vi "Test Quaternion Average.vi"(11 "Test Case In":refnum<class "03_AR.lvclass">) -> (0 "error out":errorcluster, 3 "Test Case Out":refnum<class "03_AR.lvclass">)   [LabVIEW 2020, in "test.lvlib" / "03_AR.lvclass"]
uses:
  03_AR.lvclass
  C:/Program Files (x86)/National Instruments/LabVIEW 2026/vi.lib/Astemes/LUnit/Test Case.lvclass
  ar/Quaternion.ctl
  <vilib>/Astemes/LUnit/Test Case.lvclass/Test Case.ctl
  4993e8ee-a06a-463a-9684-69129f64d5ce.vi
  <vilib>/Astemes/LUnit/Core/LUnit Test Case/Private/Append Pass Result.vi
  <vilib>/Astemes/LUnit/Core/LUnit Test Case/Private/Append Fail Result.vi
  4993e8ee-a06a-463a-9684-69129f64d5ce.vi/9c5d11cd-9439-4240-a1ee-d9baace9c924.vi
  <vilib>/Astemes/LUnit/Core/LUnit Test Case/Private/Run In UI.vi
  <vilib>/Utility/error.llb/Clear Errors.vi
  <vilib>/Utility/error.llb/Error Cluster From Error Code.vi
  ar/ar.lvlib
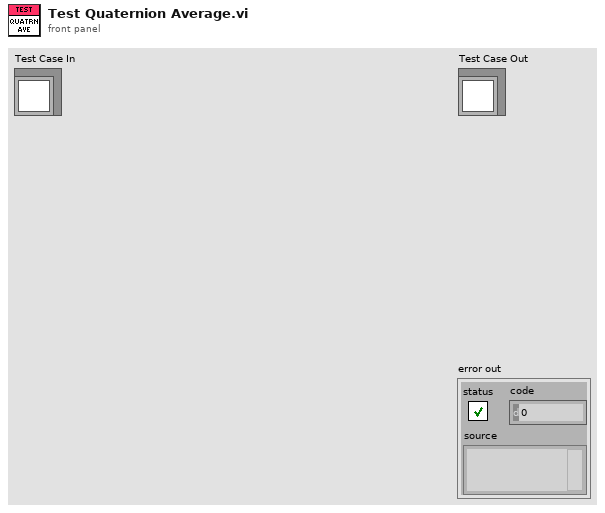
[diagram p1: front panel]
types:
  T1 = typedef "ar.lvlib/Quaternion.ctl" = cluster{"w":dbl, "x":dbl, "y":dbl, "z":dbl}
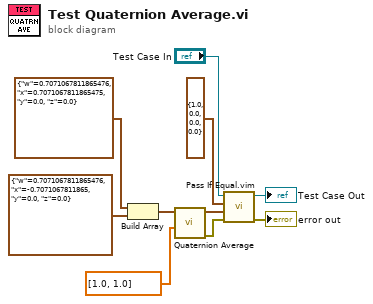
[diagram p0: block diagram]
diagram:
  n1 = Build Array(T1 {"w"=0.7071067811865476, "x"=0.7071067811865475, "y"=0.0, "z"=0.0} ("Quaternion"), T1 {"w"=0.7071067811865476, "x"=-0.7071067811865, "y"=0.0, "z"=0.0} ("Quaternion")) -> (w6:T1[])
  n2 = call "Quaternion Average.vi"("Weights (Default: Empty = equal weights)"=dbl[] [1.0, 1.0], "Quaternions"=w6) -> ("error out"=w3:errorcluster, "Average Quaternion"=w5:T1)  [unwired: 8 in]
  n3 = call "Pass If Equal.vim"("error in (no error)"=w3, "Actual"=w5, "Expected"=T1 {"w"=1.0, "x"=0.0, "y"=0.0, "z"=0.0} ("Quaternion"), "LUnit Test Case In"="Test Case In") -> ("error out"=→"error out":errorcluster, "LUnit Test Case Out"=→"Test Case Out":refnum<class "03_AR.lvclass">)  [unwired: 6 in]
